vi "Utility_Build remainder array for gaps.vi"(10 "Remainder":i32, 11 "Gap Count":i32) -> (3 "Extra gap array":i16[](array[numeric]))   [LabVIEW 2014]
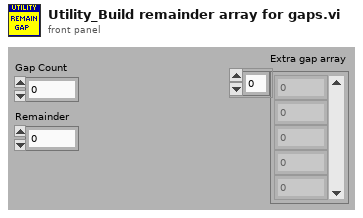
[diagram p1: front panel]
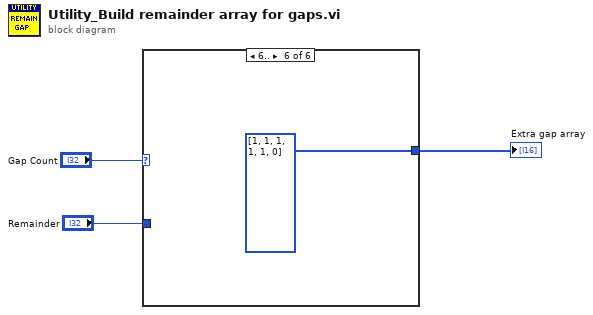
[diagram p0: block diagram]
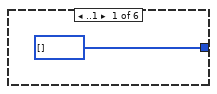
[diagram p2: hidden frame]
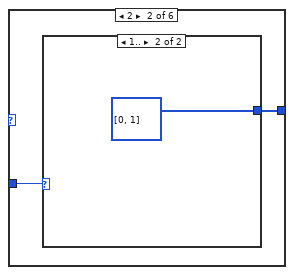
[diagram p3: hidden frame]
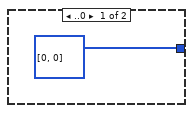
[diagram p4: hidden frame]
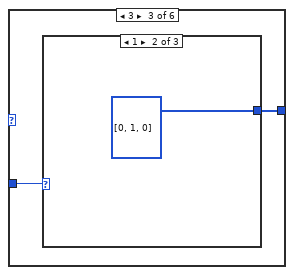
[diagram p5: hidden frame]
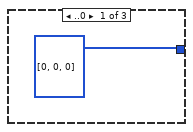
[diagram p6: hidden frame]
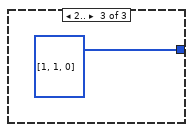
[diagram p7: hidden frame]
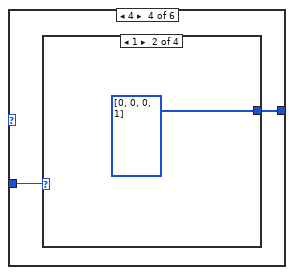
[diagram p8: hidden frame]
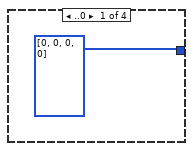
[diagram p9: hidden frame]
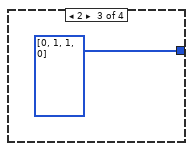
[diagram p10: hidden frame]
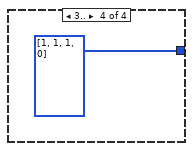
[diagram p11: hidden frame]
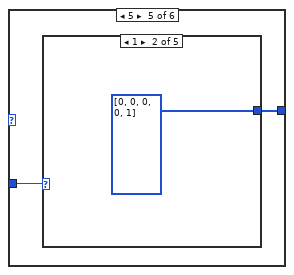
[diagram p12: hidden frame]
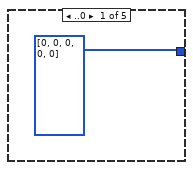
[diagram p13: hidden frame]
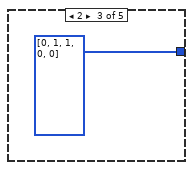
[diagram p14: hidden frame]
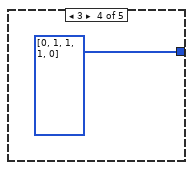
[diagram p15: hidden frame]
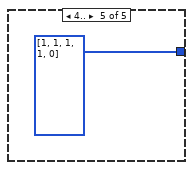
[diagram p16: hidden frame]
diagram:
  n1 = case shown="6.." "Gap Count" {
    tunnel: [i16[] [] ("Extra gap array") w6 w10 w15 w21 i16[] [1, 1, 1, 1, 1, 0] ("Extra gap array")] -> w2
    tunnel: "Remainder" -> [_ w5 w9 w14 w20 _]
    frame ..1 {
    }
    frame 2 {
      n2 = case shown="1.." w5 {
        tunnel: [i16[] [0, 0] ("Extra gap array") i16[] [0, 1] ("Extra gap array")] -> w6
        frame ..0 {
        }
        frame 1.. {
        }
      }
    }
    frame 3 {
      n3 = case shown="1" w9 {
        tunnel: [i16[] [0, 0, 0] ("Extra gap array") i16[] [0, 1, 0] ("Extra gap array") i16[] [1, 1, 0] ("Extra gap array")] -> w10
        frame ..0 {
        }
        frame 1 {
        }
        frame 2.. {
        }
      }
    }
    frame 4 {
      n4 = case shown="1" w14 {
        tunnel: [i16[] [0, 0, 0, 0] ("Extra gap array") i16[] [0, 0, 0, 1] ("Extra gap array") i16[] [0, 1, 1, 0] ("Extra gap array") i16[] [1, 1, 1, 0] ("Extra gap array")] -> w15
        frame ..0 {
        }
        frame 1 {
        }
        frame 2 {
        }
        frame 3.. {
        }
      }
    }
    frame 5 {
      n5 = case shown="1" w20 {
        tunnel: [i16[] [0, 0, 0, 0, 0] ("Extra gap array") i16[] [0, 0, 0, 0, 1] ("Extra gap array") i16[] [0, 1, 1, 0, 0] ("Extra gap array") i16[] [0, 1, 1, 1, 0] ("Extra gap array") i16[] [1, 1, 1, 1, 0] ("Extra gap array")] -> w21
        frame ..0 {
        }
        frame 1 {
        }
        frame 2 {
        }
        frame 3 {
        }
        frame 4.. {
        }
      }
    }
    frame 6.. {
    }
  }
  "Extra gap array" <- w2
